vi "Message String FGV.vi"(6 "Action":enum16{"Get String", "Set String", "Reset"}(ring), 8 "error in (no error)":errorcluster, 11 "Message String":string) -> (0 "error out":errorcluster, 3 "String out":string)   [LabVIEW 2017]
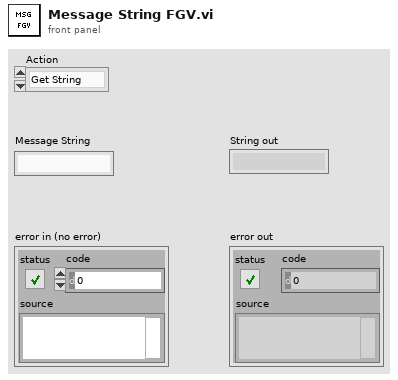
[diagram p1: front panel]
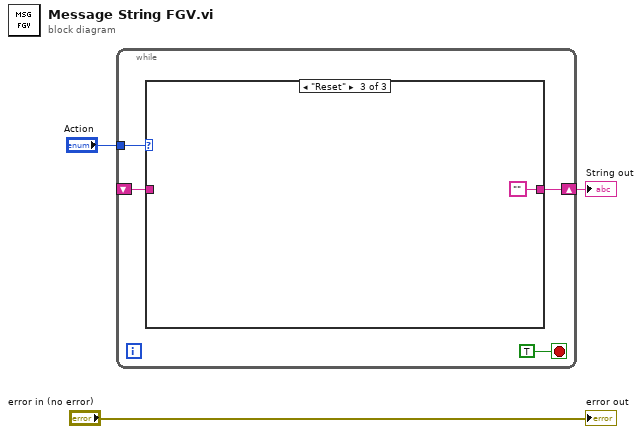
[diagram p0: block diagram]
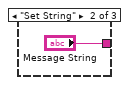
[diagram p3: hidden frame]
diagram:
  n1 = while {
    tunnel: "Action" -> [w7]
    shift-right: [w4] -> w2
    shift-left: _ -> [w5]
    stop <- TRUE stop-if-true
    n2 = case shown="\"Reset\"" w7 {
      tunnel: w5 -> [w8 _ _]
      tunnel: [w8 "Message String" ""] -> w4
      frame "Get String", Default {
      }
      frame "Set String" {
      }
      frame "Reset" {
      }
    }
  }
  "String out" <- w2
  "error out" <- "error in (no error)"
